vi "Derivative (DBL Array).vi"(2 "initialize":bool, 3 "dt":dbl=1e-09 min=1e-09 format="%.6f", 4 "initial conditions":dbl[](array[numeric]) format="%.2f", 5 "input points":dbl[](array[numeric]) format="%.2f") -> (1 "output points":dbl[](array[numeric]) format="%.2f")   [LabVIEW 2020, in "NI_AdvCtrl_continuous linear.lvlib"]
doc: "LabVIEW no longer supports this VI. You can obtain similar functionality by installing the LabVIEW Simulation Module.\n\nCalculates the derivative of a continuous signal, where the formula output(n)=(input(n)-input(n-1))/dt is used. This element is a specific transfer function with H(s)=s."
uses:
  <vilib>/addons/control/advanced/NI_AdvCtrl_continuous linear.lvlib
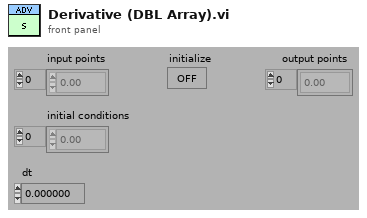
[diagram p1: front panel]
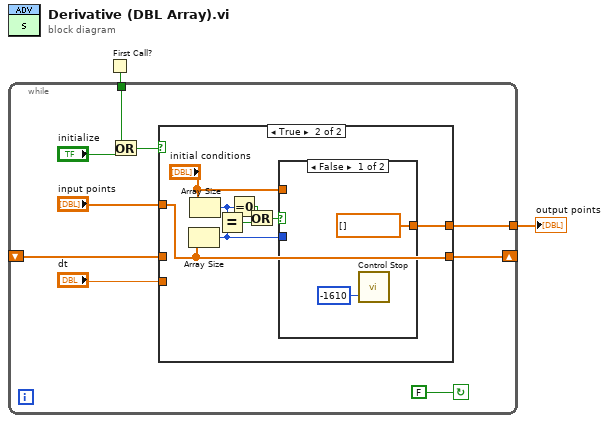
[diagram p0: block diagram]
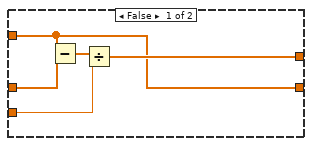
[diagram p2: hidden frame]
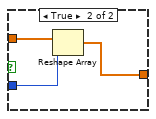
[diagram p3: hidden frame]
diagram:
  n1 = First Call?() -> (First Call?: T/F=w1:bool)
  n2 = while {
    tunnel: w1 -> [w5]
    tunnel: [w8] -> w2
    shift-left: _ -> [w10]
    shift-right: [w11] -> _
    stop <- FALSE continue-if-true
    n3 = Or(x=w5, y="initialize") -> (x .or. y?=w4:bool)
    n4 = case shown="True" w4 {
      tunnel: [w13 w24] -> w11
      tunnel: w10 -> [w16 _]
      tunnel: "input points" -> [w13 w24]
      tunnel: [w14 w22] -> w8
      tunnel: "dt" -> [w12 _]
      frame False {
        n5 = Subtract(x=w13, y=w16) -> (x-y=w15:dbl[])
        n6 = Divide(x=w15, y=w12) -> (x/y=w14:dbl[])
      }
      frame True {
        n7 = Array Size(array=w24) -> (size(s)=w17:i32)
        n8 = Array Size(array="initial conditions") -> (size(s)=w19:i32)
        n9 = Equal?(x=w19, y=w17) -> (x = y?=w20:bool)
        n10 = Equal To 0?(x=w19) -> (x = 0?=w18:bool)
        n11 = Or(x=w18, y=w20) -> (x .or. y?=w21:bool)
        n12 = case shown="False" w21 {
          tunnel: "initial conditions" -> [_ w29]
          tunnel: [dbl[] [] ("initial conditions") w28] -> w22
          tunnel: w17 -> [_ w27]
          frame False {
            n13 = call <vilib>:"Control Stop.vi"("error"=-1610) -> ()  [unwired: 2 out]
          }
          frame True {
            n14 = Reshape Array(w29, w27) -> (w28:dbl[])
          }
        }
      }
    }
  }
  "output points" <- w2
